vi "CCDWriteRoiValues.vi"(0 "CCD.lvclass":refnum<class "CCD.lvclass">, 1 "ROI":T1, 11 "error in":errorcluster) -> (4 "CCD out":refnum<class "CCD.lvclass">, 15 "error out":errorcluster)   [LabVIEW 2023]
uses:
  Classes/CCD/CCDSpectralData.ctl
  Classes/CCD/CCD.lvclass
panel:
  # "Connector Pane"
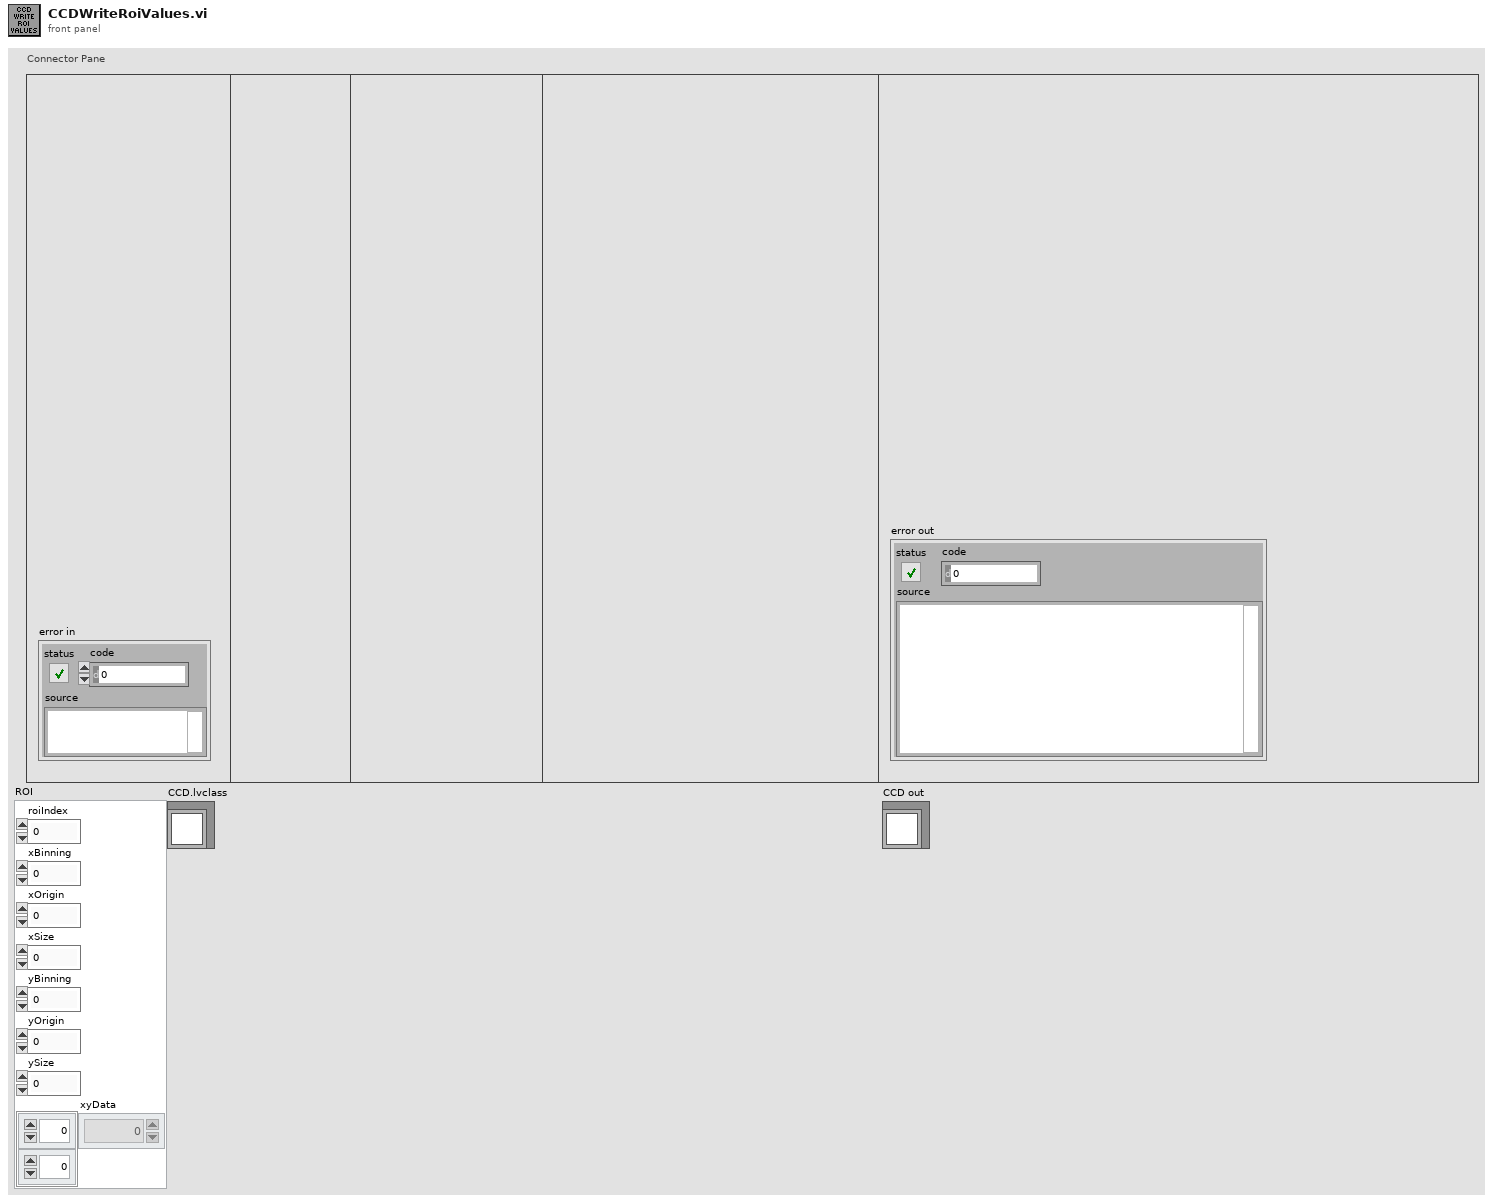
[diagram p1: front panel]
types:
  T1 = typedef "CCD.lvclass/CCDSpectralData.ctl" = cluster{"roiIndex":i32, "xBinning":i32, "xOrigin":i32, "xSize":i32, "yBinning":i32, "yOrigin":i32, "ySize":i32, "xyData":dbl[][]}
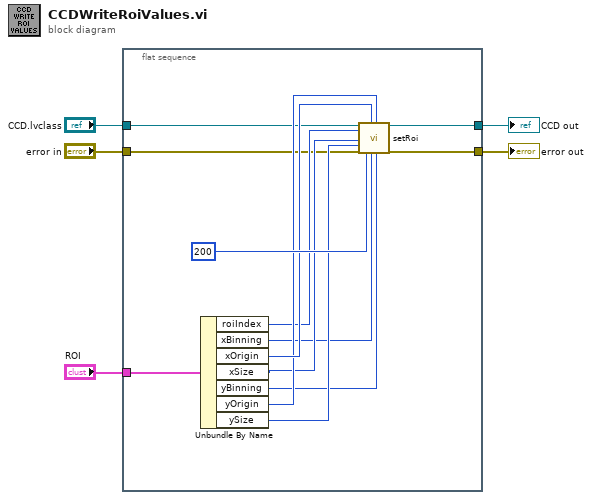
[diagram p0: block diagram]
diagram:
  n1 = flat-sequence {
    tunnel: "error in" -> [w8]
    tunnel: "CCD.lvclass" -> [w9]
    tunnel: [w6] -> w1
    tunnel: [w7] -> w5
    tunnel: "ROI" -> [w17]
    frame #0 {
      n2 = Unbundle By Name(w17) -> ("roiIndex"=w10:i32, "xBinning"=w12:i32, "xOrigin"=w16:i32, "xSize"=w14:i32, "yBinning"=w11:i32, "yOrigin"=w15:i32, "ySize"=w13:i32)
      n3 = call "setRoi.vi"("CCD in"=w9, "ROI-index"=w10, "xSize"=w14, "ySize"=w13, "error in (no error)"=w8, "Delay between send and receive [ms]"=200, "xOrigin"=w16, "xBin"=w12, "yOrigin"=w15, "yBin"=w11) -> ("CCD out"=w7:refnum<class "CCD.lvclass">, "error out"=w6:errorcluster)  [unwired: 6 in, 2 out]
    }
  }
  "error out" <- w1
  "CCD out" <- w5
